vi "Force Accuracy Test DAA.vi"(8 "error in (no error)":errorcluster, 10 "Model in":refnum<class "Model.lvclass">, 11 "Test Actuator State in":refnum<class "Test Actuator State.lvclass">) -> (0 "error out":errorcluster, 1 "Pass":bool, 2 "Model out":refnum<class "Model.lvclass">, 3 "Test Actuator State out":refnum<class "Test Actuator State.lvclass">)   [LabVIEW 2016]
uses:
  Model/Model/Model.lvclass
  Typedefs/ActuatorSetPoints.ctl
  Model/Waveforms/Waveform/Waveform.lvclass
  <vilib>/Analysis/NI_AALPro.lvlib
  <vilib>/Analysis/5stat.llb/RMS (DBL).vi
  <vilib>/Analysis/NI_AALBase.lvlib
  <vilib>/Analysis/baseanly.llb/Mean (DBL).vi
  <vilib>/platform/TimedLoop/XDataNode/XDataNode.xnode
  <vilib>/Platform/TimedLoop/XDataNode/nitl_modes.ctl
  <vilib>/Platform/TimedLoop/XDataNode/XDNodeRunTimeDep.lvlib
  <vilib>/Platform/TimedLoop/XDataNode/wakeup.ctl
  <vilib>/Platform/TimedLoop/XDataNode/timing_clust.ctl
  Test Actuator State.lvclass
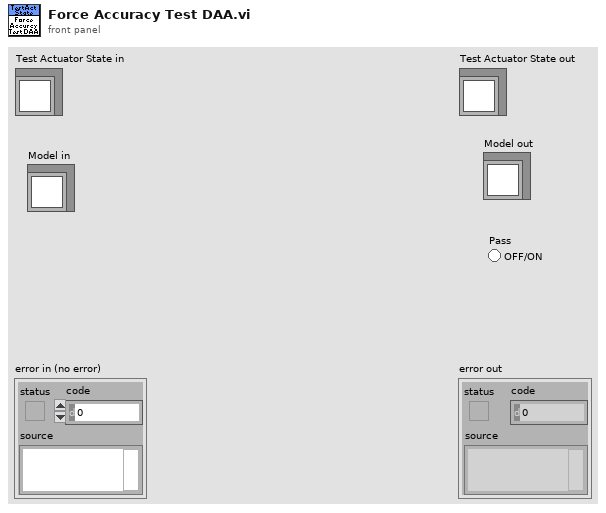
[diagram p1: front panel]
types:
  T1 = typedef "ForceAccuracyTestSettings.ctl" = cluster{"Max Force Error (N)":dbl, "Max Moment (NM)":dbl, "Process Time (s)":dbl, "Sample Time (s)":dbl, "Iterations":i32, "Amplitude (N)":dbl, "Non-Repeating Error":dbl}
  T2 = typedef "XDNodeRunTimeDep.lvlib/timing_clust.ctl" = cluster{"Expected End [f-1]":u64, "Actual End [f-1]":u64, "Finished Late? [f-1]":bool, "Expected End [i-1]":u64, "Actual End [i-1]":u64, "Finished Late? [i-1]":bool, "Expected Start [i]":u64, "Actual Start [i]":u64, "Expected Start [f]":u64, "Actual Start [f]":u64, "Source Name":string, "Structure Name":string, "Period":i64, "Deadline":i64, "Offset":i64, "Start":i64, "Priority":i32, "Timeout":i32, "Mode":T3, "Wakeup Reason":T4, "Error":errorcluster, "Source Type":string, "Secondary Source Type":string, "Global End Time":u64, "Global Start Time":u64, "Frame Duration":u64, "Iteration Duration":u64, "Assigned CPU":i32, "I/O Scan Engine Mode":u32}
  T3 = typedef "XDNodeRunTimeDep.lvlib/nitl_modes.ctl" = enum32{"No Change", "Process missed periods, maintain original phase", "Discard missed periods, maintain original phase", "Process missed periods, ignore original phase", "Discard missed periods, ignore original phase"}
  T4 = typedef "XDNodeRunTimeDep.lvlib/wakeup.ctl" = enum32{"Normal", "Aborted", "Asynchronous wakeup", "Timing source error", "Timed loop error", "Timeout"}
  T5 = typedef "ActuatorSetPoints.ctl" = cluster{"Axial Force":dbl, "Lateral Force":dbl, "FC1 Force":dbl, "FC2 Force":dbl}
  T6 = typedef "ActuatorData.ctl" = cluster{"Timestamp":dbl, "Force":dbl, "Encoder Value":i32}
  T7 = typedef "ToveyEngData.ctl" = cluster{"Timestamp":dbl, "Fx":dbl, "Fy":dbl, "Fz":dbl, "Mx":dbl, "My":dbl, "Mz":dbl}
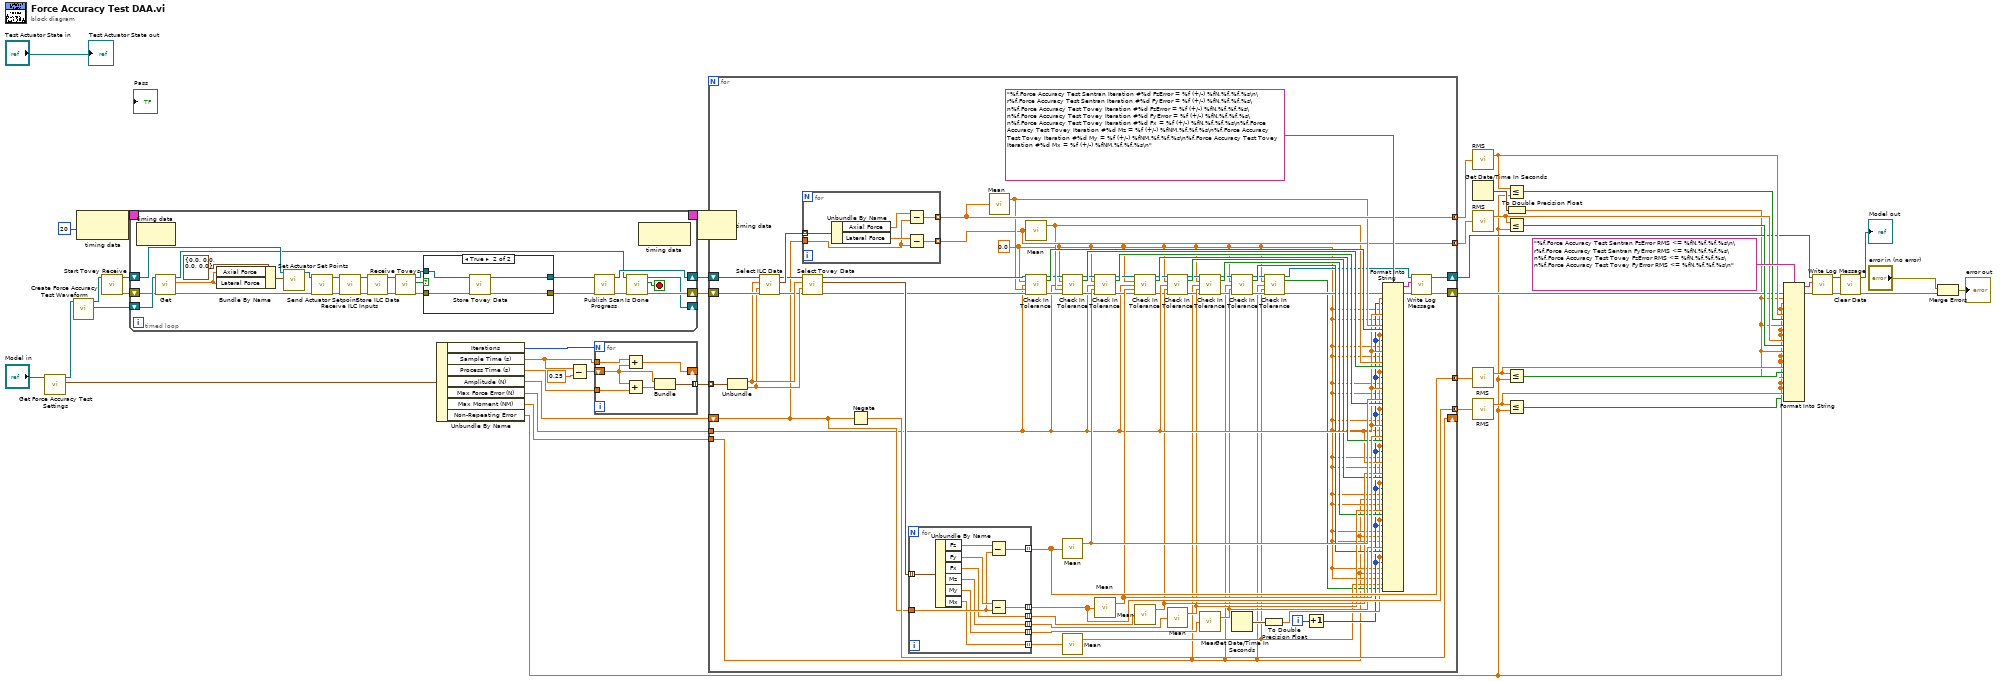
[diagram p0: block diagram]
diagram:
  n1 = call-dynamic "Get Force Accuracy Test Settings.vi"("Model in"="Model in") -> ("Force Accuracy Test Settings"=w43:T1, "Model out"=w44:refnum<class "Model.lvclass">)  [unwired: 9 in]
  n2 = call "Create Force Accuracy Test Waveform.vi"("Model in"=w44) -> ("Waveform"=w37:refnum<class "Waveform.lvclass">, "Model out"=w38:refnum<class "Model.lvclass">)  [unwired: 9 in]
  n3 = node-c288(i64 20 ("Period")) -> (w3:T2)
  n4 = call "Start Tovey Receive.vi"("Model in"=w38) -> ("error out"=w39:errorcluster, "Model out"=w40:refnum<class "Model.lvclass">)  [unwired: 9 in]
  n5 = timed-loop {
    shift-right: [w69] -> w31
    shift-left: w40 -> [w61]
    shift-right: [w52] -> w30
    shift-left: w39 -> [w55]
    shift-right: [w50] -> _
    shift-left: w37 -> [w57]
    timing: w3 -> [_]
    timing-out: [_] -> w2
    stop <- w51 stop-if-true
    n6 = node-c288() -> ()  [unwired: 1 in, 1 out]
    n7 = call-dynamic "Get.vi"("error in (no error)"=w55, "Waveform in"=w57) -> ("error out"=w54:errorcluster, "Value"=w49:dbl, "Waveform out"=w56:refnum<class "Waveform.lvclass">)  [unwired: 7 in]
    n8 = Bundle By Name(cluster=T5 {"Axial Force"=0.0, "Lateral Force"=0.0, "FC1 Force"=0.0, "FC2 Force"=0.0} ("Actuator Set Points"), "Axial Force"=w49, "Lateral Force"=w49) -> (w58:T5)
    n9 = call "Set Actuator Set Points.vi"("Actuator Set Points"=w58, "Model in"=w61) -> ("Model out"=w60:refnum<class "Model.lvclass">)  [unwired: 9 in]
    n10 = call "Send Actuator Setpoint.vi"("error in (no error)"=w54, "Model in"=w60) -> ("error out"=w71:errorcluster, "Model out"=w73:refnum<class "Model.lvclass">)  [unwired: 8 in]
    n11 = call "Receive ILC Inputs.vi"("error in (no error)"=w71, "Model in"=w73) -> ("error out"=w70:errorcluster, "Model out"=w72:refnum<class "Model.lvclass">)  [unwired: 8 in]
    n12 = call "Store ILC Data.vi"("error in (no error)"=w70, "Model in"=w72) -> ("error out"=w67:errorcluster, "Model out"=w68:refnum<class "Model.lvclass">)  [unwired: 8 in]
    n13 = call "Receive Toveys.vi"("error in (no error)"=w67, "Model in"=w68) -> ("error out"=w65:errorcluster, "Data Received"=w64:bool, "Model out"=w66:refnum<class "Model.lvclass">)  [unwired: 7 in]
    n14 = case shown="True" w64 {
      tunnel: w66 -> [w77 w81]
      tunnel: w65 -> [w76 w80]
      tunnel: [w76 w79] -> w62
      tunnel: [w77 w78] -> w63
      frame False {
      }
      frame True {
        n15 = call "Store Tovey Data.vi"("error in (no error)"=w80, "Model in"=w81) -> ("error out"=w79:errorcluster, "Model out"=w78:refnum<class "Model.lvclass">)  [unwired: 8 in]
      }
    }
    n16 = call "Publish Scan Progress.vi"("error in (no error)"=w62, "Model in"=w63) -> ("error out"=w53:errorcluster, "Model out"=w69:refnum<class "Model.lvclass">)  [unwired: 8 in]
    n17 = call-dynamic "Is Done.vi"("error in (no error)"=w53, "Waveform in"=w56) -> ("error out"=w52:errorcluster, "Is Done"=w51:bool, "Waveform out"=w50:refnum<class "Waveform.lvclass">)  [unwired: 7 in]
    n18 = node-c288() -> ()  [unwired: 1 in, 1 out]
  }
  n19 = Unbundle By Name(w43) -> ("Iterations"=w32:i32, "Sample Time (s)"=w33:dbl, "Process Time (s)"=w34:dbl, "Amplitude (N)"=w28:dbl, "Max Force Error (N)"=w23:dbl, "Max Moment (NM)"=w22:dbl, "Non-Repeating Error"=w7:dbl)
  n20 = Subtract(x=w33, y=0.25) -> (x-y=w35:dbl)
  n21 = for {
    N: w32 -> [_]
    shift-right: [w85] -> _
    shift-left: w35 -> [w83]
    tunnel: w34 -> [w87]
    tunnel: w33 -> [w86]
    tunnel: [w82] -> w29 mode=indexing
    n22 = Add(x=w86, y=w83) -> (x+y=w85:dbl)
    n23 = Add(x=w83, y=w87) -> (x+y=w84:dbl)
    n24 = Bundle(w83, w84) -> (w82:cluster{dbl, dbl})  [unwired: 1 in]
  }
  n25 = node-c288(w2) -> ()  [unwired: 1 out]
  n26 = for {
    tunnel: w29 -> [w152] mode=indexing
    shift-right: [w132] -> w12
    shift-left: w31 -> [w151]
    shift-right: [w149] -> _
    shift-left: w28 -> [w129]
    tunnel: [w139] -> w27 mode=concatenating
    tunnel: [w130] -> w26 mode=concatenating
    shift-right: [w133] -> w15
    shift-left: w30 -> [w148]
    tunnel: [w124] -> w25 mode=concatenating
    tunnel: [w119] -> w24 mode=concatenating
    tunnel: w23 -> [w113]
    tunnel: w22 -> [w88]
    i -> [w140]
    w91 = 0.0
    n27 = Unbundle(w152) -> (w146:dbl, w145:dbl)
    n28 = call "Select ILC Data.vi"("error in (no error)"=w148, "End Time"=w145, "Start Time"=w146, "Model in"=w151) -> ("error out"=w144:errorcluster, "Data"=w150:T6[], "Model out"=w147:refnum<class "Model.lvclass">)  [unwired: 4 in, 1 out]
    n29 = for {
      tunnel: w150 -> [w168] mode=indexing
      tunnel: w129 -> [w164]
      tunnel: [w166] -> w139 mode=indexing
      tunnel: [w163] -> w130 mode=indexing
      n30 = Unbundle By Name(w168) -> ("Axial Force"=w167:dbl, "Lateral Force"=w165:dbl)
      n31 = Subtract(x=w167, y=w164) -> (x-y=w166:dbl)
      n32 = Subtract(x=w165, y=w164) -> (x-y=w163:dbl)
    }
    n33 = call "Select Tovey Data.vi"("error in (no error)"=w144, "End Time"=w145, "Start Time"=w146, "Model in"=w147) -> ("error out"=w137:errorcluster, "Data"=w143:T7[], "Model out"=w138:refnum<class "Model.lvclass">)  [unwired: 4 in, 1 out]
    n34 = Negate(x=w129) -> (-x=w149:dbl)
    n35 = for {
      tunnel: w129 -> [w159]
      tunnel: [w161] -> w124 mode=indexing
      tunnel: [w158] -> w119 mode=indexing
      tunnel: [w157] -> w114 mode=indexing
      tunnel: [w156] -> w108 mode=indexing
      tunnel: [w155] -> w103 mode=indexing
      tunnel: [w154] -> w96 mode=indexing
      tunnel: w143 -> [w153] mode=indexing
      n36 = Unbundle By Name(w153) -> ("Fz"=w162:dbl, "Fy"=w160:dbl, "Fx"=w157:dbl, "Mz"=w156:dbl, "My"=w155:dbl, "Mx"=w154:dbl)
      n37 = Subtract(x=w162, y=w159) -> (x-y=w161:dbl)
      n38 = Subtract(x=w160, y=w159) -> (x-y=w158:dbl)
    }
    n39 = call-poly <vilib>:"Mean.vi"("X"=w139) -> ("mean"=w135:dbl)  [unwired: 1 out]
    n40 = call-poly <vilib>:"Mean.vi"("X"=w130) -> ("mean"=w128:dbl)  [unwired: 1 out]
    n41 = call "Check In Tolerance.vi"("Model in"=w138, "Expected"=w91, "Tolerance"=w113, "Actual"=w135, "error in (no error)"=w137) -> ("Model out"=w125:refnum<class "Model.lvclass">, "Pass"=w136:bool, "error out"=w126:errorcluster)  [unwired: 8 in]
    n42 = call "Check In Tolerance.vi"("Model in"=w125, "Expected"=w91, "Tolerance"=w113, "Actual"=w128, "error in (no error)"=w126) -> ("Model out"=w122:refnum<class "Model.lvclass">, "Pass"=w127:bool, "error out"=w121:errorcluster)  [unwired: 8 in]
    n43 = call-poly <vilib>:"Mean.vi"("X"=w124) -> ("mean"=w123:dbl)  [unwired: 1 out]
    n44 = call-poly <vilib>:"Mean.vi"("X"=w96) -> ("mean"=w90:dbl)  [unwired: 1 out]
    n45 = call "Check In Tolerance.vi"("Model in"=w122, "Expected"=w91, "Tolerance"=w113, "Actual"=w123, "error in (no error)"=w121) -> ("Model out"=w116:refnum<class "Model.lvclass">, "Pass"=w120:bool, "error out"=w115:errorcluster)  [unwired: 8 in]
    n46 = call-poly <vilib>:"Mean.vi"("X"=w119) -> ("mean"=w118:dbl)  [unwired: 1 out]
    n47 = call "Check In Tolerance.vi"("Model in"=w116, "Expected"=w91, "Tolerance"=w113, "Actual"=w118, "error in (no error)"=w115) -> ("Model out"=w110:refnum<class "Model.lvclass">, "Pass"=w117:bool, "error out"=w109:errorcluster)  [unwired: 8 in]
    n48 = call-poly <vilib>:"Mean.vi"("X"=w114) -> ("mean"=w112:dbl)  [unwired: 1 out]
    n49 = call "Check In Tolerance.vi"("Model in"=w110, "Expected"=w91, "Tolerance"=w113, "Actual"=w112, "error in (no error)"=w109) -> ("Model out"=w105:refnum<class "Model.lvclass">, "Pass"=w111:bool, "error out"=w104:errorcluster)  [unwired: 8 in]
    n50 = call-poly <vilib>:"Mean.vi"("X"=w108) -> ("mean"=w107:dbl)  [unwired: 1 out]
    n51 = call "Check In Tolerance.vi"("Model in"=w105, "Expected"=w91, "Tolerance"=w88, "Actual"=w107, "error in (no error)"=w104) -> ("Model out"=w100:refnum<class "Model.lvclass">, "Pass"=w106:bool, "error out"=w99:errorcluster)  [unwired: 8 in]
    n52 = call-poly <vilib>:"Mean.vi"("X"=w103) -> ("mean"=w102:dbl)  [unwired: 1 out]
    n53 = call "Check In Tolerance.vi"("Model in"=w100, "Expected"=w91, "Tolerance"=w88, "Actual"=w102, "error in (no error)"=w99) -> ("Model out"=w95:refnum<class "Model.lvclass">, "Pass"=w101:bool, "error out"=w93:errorcluster)  [unwired: 8 in]
    n54 = Get Date/Time In Seconds() -> (seconds since 1Jan1904=w141:timestamp)
    n55 = To Double Precision Float(number=w141) -> (double precision float=w98:dbl)
    n56 = call "Check In Tolerance.vi"("Model in"=w95, "Expected"=w91, "Tolerance"=w88, "Actual"=w90, "error in (no error)"=w93) -> ("Model out"=w94:refnum<class "Model.lvclass">, "Pass"=w89:bool, "error out"=w92:errorcluster)  [unwired: 8 in]
    n57 = Increment(x=w140) -> (x+1=w97:i32)
    n58 = Format Into String(format string="%f,Force Accuracy Test Sentran Iteration #%d FzError = %f (+/-) %fN,%f,%f,%s\n\r%f,Force Accuracy Test Sentran Iteration #%d FyError = %f (+/-) %fN,%f,%f,%s\n%f,Force Accuracy Test Tovey Iteration #%d FzError = %f (+/-) %fN,%f,%f,%s\n%f,Force Accuracy Test Tovey Iteration #%d FyError = %f (+/-) %fN,%f,%f,%s\n%f,Force Accuracy Test Tovey Iteration #%d Fx = %f (+/-) %fN,%f,%f,%s\n%f,Force Accuracy Test Tovey Iteration #%d Mz = %f (+/-) %fNM,%f,%f,%s\n%f,Force Accuracy Test Tovey Iteration #%d My = %f (+/-) %fNM,%f,%f,%s\n%f,Force Accuracy Test Tovey Iteration #%d Mx = %f (+/-) %fNM,%f,%f,%s\n", error in=w92, w98, w97, w91, w113, w91, w135, w136, w98, w97, w91, w113, w91, w128, w127, w98, w97, w91, w113, w91, w123, w120, w98, w97, w91, w113, w91, w118, w117, w98, w97, w91, w113, w91, w112, w111, w98, w97, w91, w88, w91, w107, w106, w98, w97, w91, w88, w91, w102, w101, w98, w97, w91, w88, w91, w90, w89) -> (resulting string=w131:string, error out=w134:errorcluster)  [unwired: 1 in]
    n59 = call "Write Log Message.vi"("error in (no error)"=w134, "Message"=w131, "Model in"=w94) -> ("error out"=w133:errorcluster, "Model out"=w132:refnum<class "Model.lvclass">)  [unwired: 7 in]
  }
  n60 = call-poly <vilib>:"RMS.vi"("X"=w27) -> ("rms value"=w19:dbl)  [unwired: 1 out]
  n61 = Get Date/Time In Seconds() -> (seconds since 1Jan1904=w20:timestamp)
  n62 = call-poly <vilib>:"RMS.vi"("X"=w26) -> ("rms value"=w17:dbl)  [unwired: 1 out]
  n63 = call-poly <vilib>:"RMS.vi"("X"=w25) -> ("rms value"=w11:dbl)  [unwired: 1 out]
  n64 = call-poly <vilib>:"RMS.vi"("X"=w24) -> ("rms value"=w8:dbl)  [unwired: 1 out]
  n65 = Less Or Equal?(x=w19, y=w7) -> (x <= y?=w18:bool)
  n66 = Less Or Equal?(x=w17, y=w7) -> (x <= y?=w16:bool)
  n67 = Less Or Equal?(x=w11, y=w7) -> (x <= y?=w10:bool)
  n68 = Less Or Equal?(x=w8, y=w7) -> (x <= y?=w6:bool)
  n69 = To Double Precision Float(number=w20) -> (double precision float=w9:dbl)
  n70 = Format Into String(format string="%f,Force Accuracy Test Sentran FzError RMS <= %fN,%f,%f,%s\n\r%f,Force Accuracy Test Sentran FyError RMS <= %fN,%f,%f,%s\n%f,Force Accuracy Test Tovey FzError RMS <= %fN,%f,%f,%s\n%f,Force Accuracy Test Tovey FyError RMS <= %fN,%f,%f,%s\n", error in=w15, w9, w7, w7, w19, w18, w9, w7, w7, w17, w16, w9, w7, w7, w11, w10, w9, w7, w7, w8, w6) -> (resulting string=w13:string, error out=w14:errorcluster)  [unwired: 1 in]
  n71 = call "Write Log Message.vi"("error in (no error)"=w14, "Message"=w13, "Model in"=w12) -> ("error out"=w5:errorcluster, "Model out"=w4:refnum<class "Model.lvclass">)  [unwired: 7 in]
  n72 = call "Clear Data.vi"("error in (no error)"=w5, "Model in"=w4) -> ("error out"=w42:errorcluster, "Model out"=→"Model out":refnum<class "Model.lvclass">)  [unwired: 8 in]
  n73 = Merge Errors("error in (no error)", w42) -> (→"error out":errorcluster)
  "Test Actuator State out" <- "Test Actuator State in"
